vi "InitializeMain.vi"(8 "error in":errorcluster, 10 "Settings (Clamp (Rake))":T3, 11 "Hardware Info":T4={"LED Channel"="MyDigitalOutTask", "Force Sensor Channel"="Dev2/ai7", "Servo Channel"="MyPulseOutputTask", "Camera Selector"="cam5", "Camera Freq"=30.0, "FS Freq"=30.0, "Servo Freq"=30.0, "Color Pane"=0} {"Color Pane" items=["Blue", "Red", "Green", "Saturation", "Value", "Intensity", "Luminance", "Hue", ""]}) -> (0 "error out":errorcluster, 2 "New Image":T5, 3 "Task Output":T2)   [LabVIEW 2020]
uses:
  <vilib>/vision/Image Controls.llb/IMAQ Image.ctl
  Controls/HWchannels.ctl
  <vilib>/userdefined/High Color/IMAQdx.ctl
  <vilib>/DAQmx/create/channels.llb/DAQmx Create Channel (AI-Voltage-Basic).vi
  <vilib>/DAQmx/configure/timing.llb/DAQmx Timing (Sample Clock).vi
  <vilib>/vision/driver/NI_Vision_Acquisition_Software.lvlib
panel:
  # "Channel"
  # "Frequency (Hz)"
  # "Force Sensor:"
  # "Servo:"
  # "LED:"
  # "N/A"
  # "Camera:"
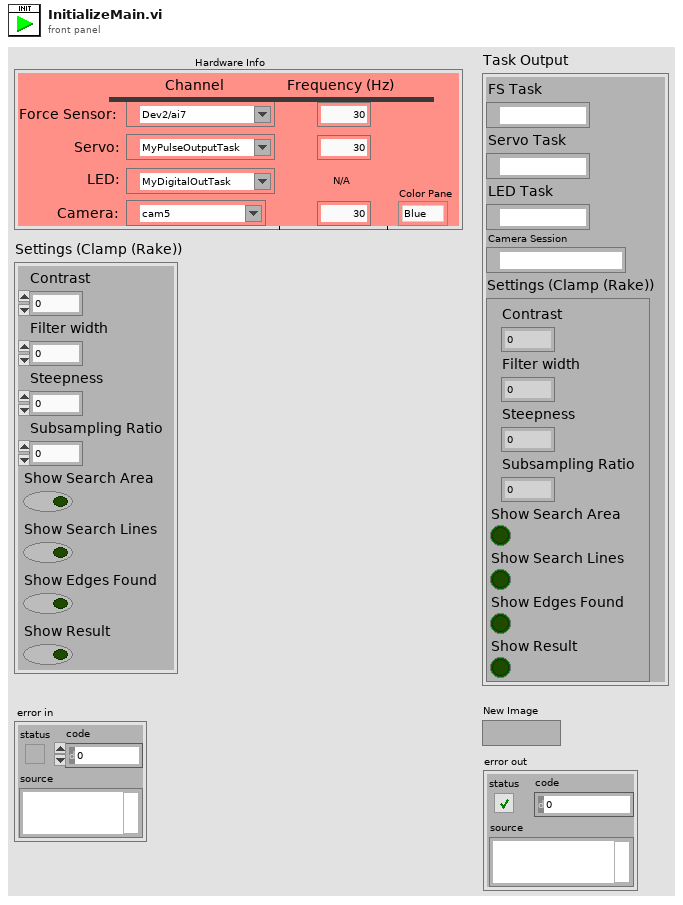
[diagram p1: front panel]
types:
  T1 = typedef "IMAQdx.ctl" = refnum<k21>
  T2 = cluster{"FS Task":refnum<k21>, "Servo Task":refnum<k21>, "LED Task":refnum<k21>, "Camera Session":T1, "Settings (Clamp (Rake))":cluster{"Contrast":i32, "Filter width":i32, "Steepness":i32, "Subsampling Ratio":u32, "Show Search Area":bool, "Show Search Lines":bool, "Show Edges Found":bool, "Show Result":bool}}
  T3 = cluster{"Contrast":i32, "Filter width":i32, "Steepness":i32, "Subsampling Ratio":u32, "Show Search Area":bool, "Show Search Lines":bool, "Show Edges Found":bool, "Show Result":bool}
  T4 = typedef "HWchannels.ctl" = cluster{"LED Channel":refnum<k21>, "Force Sensor Channel":tag, "Servo Channel":refnum<k21>, "Camera Selector":T1, "Camera Freq":dbl, "FS Freq":dbl, "Servo Freq":dbl, "Color Pane":i32}
  T5 = typedef "IMAQ Image.ctl" = refnum<image>
  T6 = typedef "Image Type" = u32
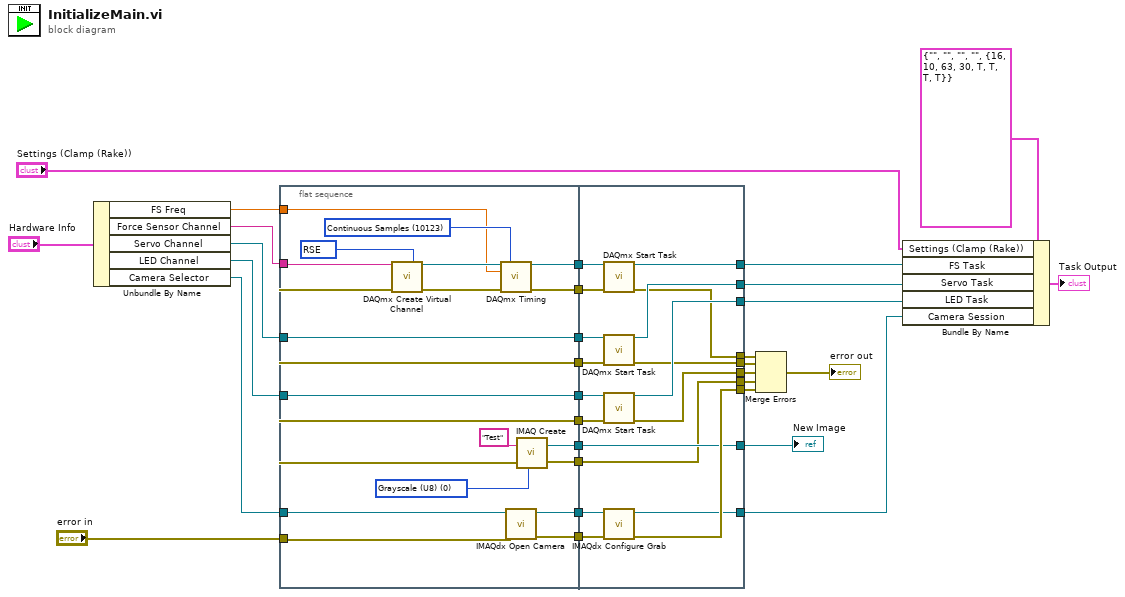
[diagram p0: block diagram]
diagram:
  n1 = Unbundle By Name("Hardware Info") -> ("FS Freq"=w27:dbl, "Force Sensor Channel"=w14:tag, "Servo Channel"=w13:refnum<k21>, "LED Channel"=w12:refnum<k21>, "Camera Selector"=w8:T1)
  n2 = flat-sequence {
    tunnel: w8 -> [w43]
    tunnel: [w42] -> w31
    tunnel: [w41] -> w30
    tunnel: [w40] -> w29
    tunnel: [w39] -> w28
    tunnel: w27 -> [w38]
    tunnel: "error in" -> [w32]
    tunnel: [w37] -> w21
    tunnel: [w36] -> w18
    tunnel: [w34] -> w16
    tunnel: [w33] -> w15
    tunnel: w14 -> [w35]
    tunnel: w13 -> [w34]
    tunnel: w12 -> [w33]
    tunnel: [w32] -> w6
    tunnel: [w32] -> w5
    tunnel: w31 -> [w67]
    tunnel: w30 -> [w66]
    tunnel: w29 -> [w65]
    tunnel: w28 -> [w64]
    tunnel: [w63] -> w11
    tunnel: [w62] -> w10
    tunnel: [w61] -> w9
    tunnel: [w60] -> w25
    tunnel: [w59] -> w24
    tunnel: [w58] -> w23
    tunnel: [w57] -> w19
    tunnel: [w56] -> w7
    tunnel: w21 -> [w55]
    tunnel: [w55] -> w20
    tunnel: w18 -> [w54]
    tunnel: [w54] -> w17
    tunnel: w16 -> [w53]
    tunnel: w15 -> [w52]
    tunnel: w6 -> [w51]
    tunnel: w5 -> [w50]
    frame #0 {
      w44 = T6 0 items=["Grayscale (U8)", "Grayscale (I16)", "Grayscale (SGL)", "Complex (CSG)", "RGB (U32)", "HSL (U32)", "RGB (U64)", "Grayscale (U16)"] ("Image Type")
      w47 = 10083 items=["Default"=-1, "RSE"=10083, "NRSE"=10078, "Differential"=10106, "Pseudodifferential"=12529] ("input terminal configuration")
      w46 = 10123 items=["Finite Samples"=10178, "Continuous Samples"=10123, "Hardware Timed Single Point"=12522] ("sample mode")
      n3 = call-poly <vilib>:"DAQmx Create Virtual Channel.vi"("input terminal configuration"=w47, "physical channels"=w35, "error in"=w32) -> ("task out"=w48:refnum<k21>, "error out"=w49:errorcluster)  [unwired: 11 in]
      n4 = call-poly <vilib>:"DAQmx Timing.vi"("task/channels in"=w48, "sample mode"=w46, "rate"=w38, "error in"=w49) -> ("task out"=w40:refnum<k21>, "error out"=w39:errorcluster)  [unwired: 10 in]
      n5 = call <vilib>:"IMAQdx Open Camera.vi"("error in"=w32, "Session In"=w43) -> ("error out"=w42:errorcluster, "Session Out"=w41:T1)  [unwired: 8 in]
      n6 = call "IMAQ Create"("Image Name"="Test", "Image Type"=w44, "error in (no error)"=w32) -> ("New Image"=w37:T5, "error out"=w36:errorcluster)  [unwired: 2 in]
    }
    frame #1 {
      n7 = call <vilib>:"DAQmx Start Task.vi"("task/channels in"=w65, "error in"=w64) -> ("task out"=w63:refnum<k21>, "error out"=w60:errorcluster)  [unwired: 12 in]
      n8 = call <vilib>:"DAQmx Start Task.vi"("task/channels in"=w53, "error in"=w51) -> ("task out"=w62:refnum<k21>, "error out"=w59:errorcluster)  [unwired: 12 in]
      n9 = call <vilib>:"DAQmx Start Task.vi"("task/channels in"=w52, "error in"=w50) -> ("task out"=w61:refnum<k21>, "error out"=w58:errorcluster)  [unwired: 12 in]
      n10 = call <vilib>:"IMAQdx Configure Grab.vi"("error in"=w67, "Session In"=w66) -> ("error out"=w57:errorcluster, "Session Out"=w56:T1)  [unwired: 8 in]
    }
  }
  n11 = Merge Errors(w25, w24, w23, w17, w19) -> (→"error out":errorcluster)
  n12 = Bundle By Name(cluster=T2 {"FS Task"="", "Servo Task"="", "LED Task"="", "Camera Session"="", "Settings (Clamp (Rake))"={"Contrast"=16, "Filter width"=10, "Steepness"=63, "Subsampling Ratio"=30, "Show Search Area"=TRUE, "Show Search Lines"=TRUE, "Show Edges Found"=TRUE, "Show Result"=TRUE}}, "Settings (Clamp (Rake))"="Settings (Clamp (Rake))", "FS Task"=w11, "Servo Task"=w10, "LED Task"=w9, "Camera Session"=w7) -> (→"Task Output":T2)
  "New Image" <- w20
